vi "CreateWaypoint.vi"(4 "Use Default?":bool, 6 "Default Altitude":dbl=5.0 caption="m", 7 "Altitude":dbl caption="m", 10 "Coordinates":string, 11 "Type":u16(ring) items=["Way Point", "Take Off", "Loiter", "Land", "Change Heading"]) -> (3 "Waypoint":T1 {"EW" items=["E", "W"]; "LonS" format="%#.1f"; "NS" items=["N", "S"]; "LatS" format="%#.1f"})   [LabVIEW 2010]
uses:
  Waypoint.ctl
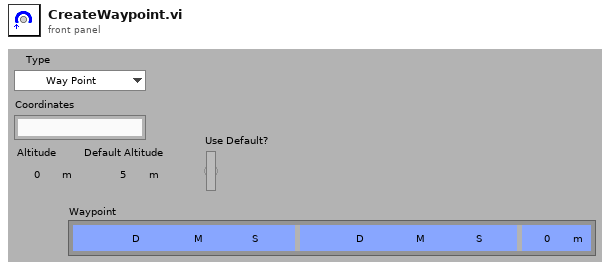
[diagram p1: front panel]
types:
  T1 = typedef "Waypoint.ctl" = cluster{"LatD":dbl, "LatM":dbl, "LatS":dbl, "LonD":dbl, "LonM":dbl, "LonS":dbl, "Alt":dbl, "NS":u16, "EW":u16}
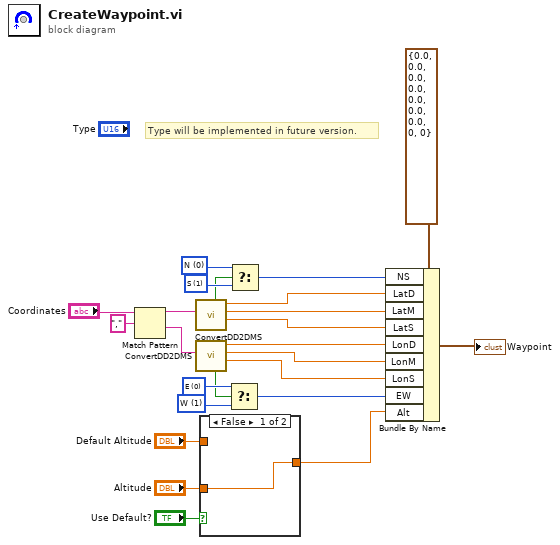
[diagram p0: block diagram]
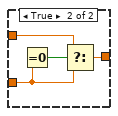
[diagram p2: hidden frame]
diagram:
  w14 = u16 1 items=["E", "W"] ("EW")
  w17 = u16 1 items=["N", "S"] ("NS")
  w15 = u16 0 items=["E", "W"] ("EW")
  w18 = u16 0 items=["N", "S"] ("NS")
  # "Type will be implemented in future version."
  n1 = Match Pattern(string="Coordinates", regular expression=",") -> (before substring=w22:string, after substring=w21:string)  [unwired: 1 in, 2 out]
  n2 = call "ConvertDD2DMS.vi"("Decimal String"=w22) -> ("Seconds"=w8:dbl, "Minutes"=w9:dbl, "Degrees"=w10:dbl, "NE?"=w16:bool)  [unwired: 6 in, 1 out]
  n3 = call "ConvertDD2DMS.vi"("Decimal String"=w21) -> ("Seconds"=w5:dbl, "Minutes"=w6:dbl, "Degrees"=w7:dbl, "NE?"=w13:bool)  [unwired: 6 in, 1 out]
  n4 = case shown="False" "Use Default?" {
    tunnel: "Altitude" -> [w25 w28]
    tunnel: "Default Altitude" -> [_ w27]
    tunnel: [w25 w26] -> w2
    frame False {
    }
    frame True {
      n5 = Equal To 0?(x=w28) -> (x = 0?=w29:bool)
      n6 = Select(t=w27, s=w29, f=w28) -> (s? t:f=w26:dbl)
    }
  }
  n7 = Select(t=w15, s=w13, f=w14) -> (s? t:f=w12:u16)
  n8 = Select(t=w18, s=w16, f=w17) -> (s? t:f=w11:u16)
  n9 = Bundle By Name(cluster=T1 {"LatD"=0.0, "LatM"=0.0, "LatS"=0.0, "LonD"=0.0, "LonM"=0.0, "LonS"=0.0, "Alt"=0.0, "NS"=0, "EW"=0} ("Waypoint"), "NS"=w11, "LatD"=w10, "LatM"=w9, "LatS"=w8, "LonD"=w7, "LonM"=w6, "LonS"=w5, "EW"=w12, "Alt"=w2) -> (→"Waypoint":T1)
